vi "LSI336Data_measure.vi"(0 "LSI336Data in":refnum<class "LSI336Data.lvclass">, 5 "MeasurementIndex":i32, 11 "error in (no error)":errorcluster, 13 "save every ... measurements":i32) -> (1 "Active?":bool[](array[boolean]), 3 "TimeMeasuremeent":timestamp, 4 "LSI336Data out":refnum<class "LSI336Data.lvclass">, 6 "LastData":dbl[](array[numeric]), 8 "LastMeasurementConfig":T1(array[cluster]), 10 "DataArray":dbl[][](array[numeric]), 12 "Status":u16(ring)=2 items=["Initialized", "Ready", "Measuring", "Terminated"], 14 "TimeArray":timestamp[](array[timestamp]), 15 "error out":errorcluster)   [LabVIEW 2020, in "LSI336Data.lvclass"]
uses:
  LSI336Data.lvclass
  LSI336Data.lvclass/LSI336Data.ctl
  istr.lib/Lake Shore 336/Public/Data/Sensor Data (Single Reading).vi
  istr.lib/Lake Shore 336/Lake Shore 336.lvlib
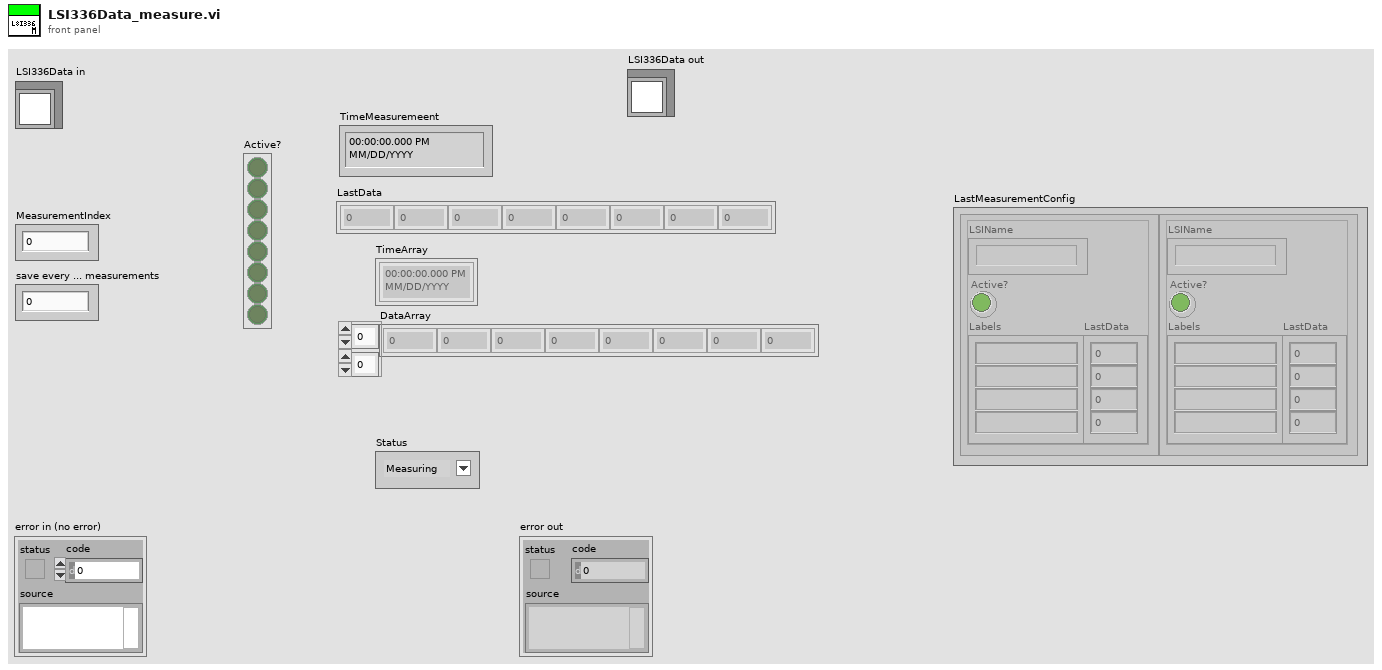
[diagram p1: front panel]
types:
  T1 = cluster{"LSIName":string, "Active?":bool, "LastData":dbl[], "Labels":string[]}[]
  T2 = cluster{"LSIName":string, "Labels":string[], "SensorLocations":enum16{"N.C.", "T3He1-1", "T3He1-2", "T3He1-3", "T3He1-4", "T3He2-1", "T3He2-2", "T3He3", "T3He4", "T3He5", "T3He6-1", "T3He6-2", "T3He7-1", "T3He7-2", "T3He8", "T3He9", "T3He10", "T4He1", "T4He2-1", "T4He2-2", "T4He3-1", "T4He3-2", "T4He3-3", "T4He3-4", "T4He4", "T4He5", "T4He6", "T4He7", "T4He8", "T4He9", "T4He10", "T1K1", "T1K2", "T1K3-1", "T1K3-2", "T1K4", "T1K5", "T1K6", "TIP1", "TIP2", "TIP3", "TIP4", "TIP5", "TIP6", "TIP7", "TTH1", "TTH2", "TTH3", "TTH4"}[], "Active?":bool, "VISA res. name":refnum<visa-resource-name>}[]
  T3 = cluster{"LSIName":string, "Labels":string[], "SensorLocations":enum16{"N.C.", "T3He1-1", "T3He1-2", "T3He1-3", "T3He1-4", "T3He2-1", "T3He2-2", "T3He3", "T3He4", "T3He5", "T3He6-1", "T3He6-2", "T3He7-1", "T3He7-2", "T3He8", "T3He9", "T3He10", "T4He1", "T4He2-1", "T4He2-2", "T4He3-1", "T4He3-2", "T4He3-3", "T4He3-4", "T4He4", "T4He5", "T4He6", "T4He7", "T4He8", "T4He9", "T4He10", "T1K1", "T1K2", "T1K3-1", "T1K3-2", "T1K4", "T1K5", "T1K6", "TIP1", "TIP2", "TIP3", "TIP4", "TIP5", "TIP6", "TIP7", "TTH1", "TTH2", "TTH3", "TTH4"}[], "Active?":bool, "VISA res. name":refnum<visa-resource-name>}
  T4 = cluster{"LSIName":string, "Active?":bool, dbl[], "Labels":string[]}
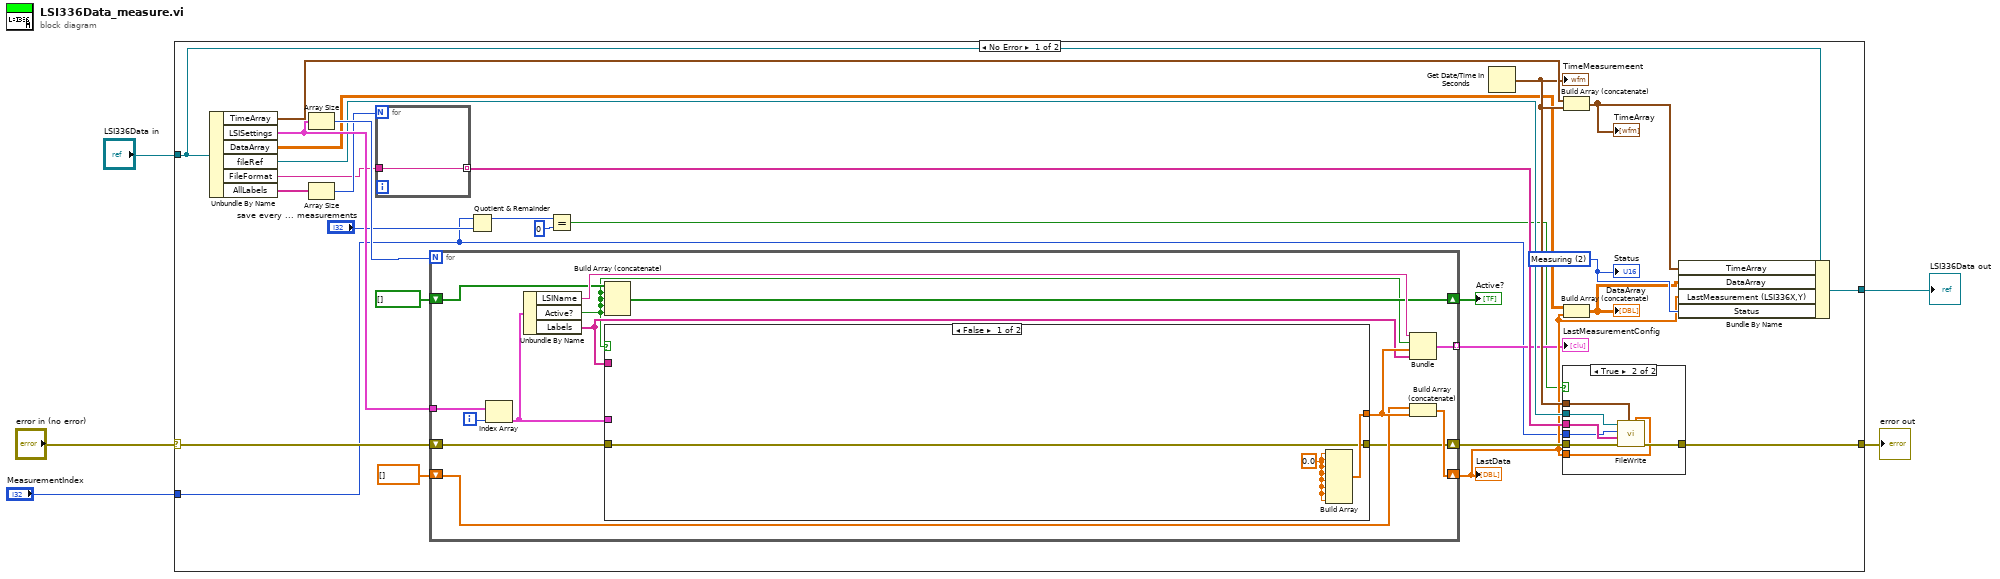
[diagram p0: block diagram]
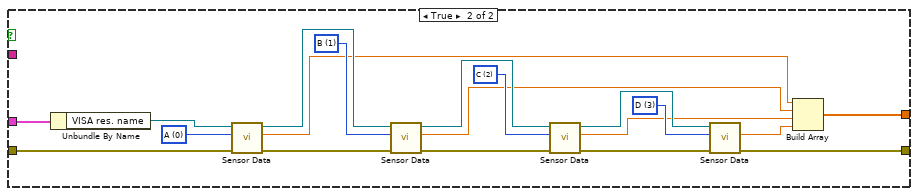
[diagram p3: hidden frame]
diagram:
  n1 = case shown="No Error" "error in (no error)" {
    selector: "error in (no error)" -> [w31 w80]
    tunnel: [w22 w80] -> w4
    tunnel: [w18 w79] -> w2
    tunnel: "LSI336Data in" -> [w19 w79]
    tunnel: "MeasurementIndex" -> [w9 _]
    frame No Error {
      w20 = u16 2 items=["Initialized", "Ready", "Measuring", "Terminated"] ("Status")
      n2 = Unbundle By Name(w19) -> ("TimeArray"=w17:timestamp[], "LSISettings"=w32:T2, "DataArray"=w15:dbl[][], "fileRef"=w24:refnum<file>, "FileFormat"=w26:string, "AllLabels"=w28:string[])
      n3 = Array Size(array=w32) -> (size(s)=w33:i32)
      n4 = Array Size(array=w28) -> (size(s)=w27:i32)
      n5 = for {
        N: w27 -> [_]
        tunnel: w26 -> [w42]
        tunnel: [w42] -> w25 mode=indexing
      }
      n6 = for {
        N: w33 -> [_]
        tunnel: w32 -> [w56]
        tunnel: [w54] -> w11 mode=indexing
        shift-right: [w52] -> w14
        shift-left: dbl[] [] -> [w51]
        shift-right: [w47] -> w21
        shift-left: bool[] [] -> [w46]
        shift-right: [w43] -> w23
        shift-left: w31 -> [w44]
        i -> [w50]
        n7 = Index Array(array=w56, index=w50) -> (element=w49:T3)
        n8 = Unbundle By Name(w49) -> ("LSIName"=w55:string, "Active?"=w45:bool, "Labels"=w48:string[])
        n9 = Build Array (concatenate)(w46, w45, w45, w45, w45) -> (w47:bool[])
        n10 = case shown="False" w45 {
          tunnel: [w58 w60] -> w53
          tunnel: w49 -> [_ w78]
          tunnel: w48 -> [_ _]
          tunnel: w44 -> [w57 w66]
          tunnel: [w57 w65] -> w43
          frame False {
            w59 = 0.0
            n11 = Build Array(w59, w59, w59, w59, w59, w59, w59, w59) -> (w58:dbl[])
          }
          frame True {
            w73 = u16 3 items=["A", "B", "C", "D"] ("Input (0:A)")
            w75 = u16 2 items=["A", "B", "C", "D"] ("Input (0:A)")
            w76 = u16 1 items=["A", "B", "C", "D"] ("Input (0:A)")
            w77 = u16 0 items=["A", "B", "C", "D"] ("Input (0:A)")
            n12 = Unbundle By Name(w78) -> ("VISA res. name"=w74:refnum<visa-resource-name>)
            n13 = call-poly "Sensor Data.vi"("error in (no error)"=w66, "Input (0:A)"=w77, "VISA resource name"=w74) -> ("error out"=w67:errorcluster, "Sensor Data"=w64:dbl, "VISA resource name out"=w72:refnum<visa-resource-name>)  [unwired: 6 in]
            n14 = call-poly "Sensor Data.vi"("error in (no error)"=w67, "Input (0:A)"=w76, "VISA resource name"=w72) -> ("error out"=w68:errorcluster, "Sensor Data"=w63:dbl, "VISA resource name out"=w71:refnum<visa-resource-name>)  [unwired: 6 in]
            n15 = call-poly "Sensor Data.vi"("error in (no error)"=w68, "Input (0:A)"=w75, "VISA resource name"=w71) -> ("error out"=w69:errorcluster, "Sensor Data"=w62:dbl, "VISA resource name out"=w70:refnum<visa-resource-name>)  [unwired: 6 in]
            n16 = call-poly "Sensor Data.vi"("error in (no error)"=w69, "Input (0:A)"=w73, "VISA resource name"=w70) -> ("error out"=w65:errorcluster, "Sensor Data"=w61:dbl)  [unwired: 6 in, 1 out]
            n17 = Build Array(w64, w63, w62, w61) -> (w60:dbl[])
          }
        }
        n18 = Bundle("LSIName"=w55, "Active?"=w45, w53, "Labels"=w48) -> (w54:T4)  [unwired: 1 in]
        n19 = Build Array (concatenate)(w51, w53) -> (w52:dbl[])
      }
      "Active?" <- w21
      "LastData" <- w14
      "LastMeasurementConfig" <- w11
      n20 = Quotient & Remainder(x=w9, y="save every ... measurements") -> (x-y*floor(x/y)=w8:i32)  [unwired: 1 out]
      n21 = Equal?(x=w8, y=0) -> (x = y?=w6:bool)
      n22 = Get Date/Time In Seconds() -> (seconds since 1Jan1904=w16:timestamp)
      "TimeMeasuremeent" <- w16
      n23 = case shown="True" w6 {
        tunnel: w25 -> [_ w41]
        tunnel: w24 -> [_ w40]
        tunnel: w9 -> [_ w39]
        tunnel: w23 -> [w34 w38]
        tunnel: [w34 w37] -> w22
        tunnel: w16 -> [_ w36]
        tunnel: w14 -> [_ w35]
        frame False {
        }
        frame True {
          n24 = call "FileWrite.vi"("DataArray"=w35, "Time Stamp"=w36, "Error In"=w38, "FileFormat"=w41, "Index"=w39, "refnum in"=w40) -> ("Error Out"=w37:errorcluster)  [unwired: 4 in, 1 out]
        }
      }
      n25 = Build Array (concatenate)(w17, w16) -> (w13:timestamp[])
      "TimeArray" <- w13
      n26 = Build Array (concatenate)(w15, w14) -> (w12:dbl[][])
      "DataArray" <- w12
      n27 = Bundle By Name(cluster=w19, "TimeArray"=w13, "DataArray"=w12, "LastMeasurement (LSI336X,Y)"=w14, "Status"=w20) -> (w18:refnum<class "LSI336Data.lvclass">)
      "Status" <- w20
    }
    frame Error {
    }
  }
  "error out" <- w4
  "LSI336Data out" <- w2
